vi "Helper - Find All Substring Locations.vi"(10 "search string":string, 11 "input string":string) -> (3 "Locations":i32[](array[numeric]))   [LabVIEW 2011]
doc: "Finds ALL instances of the search string in the input string and outputs the locations in an array."
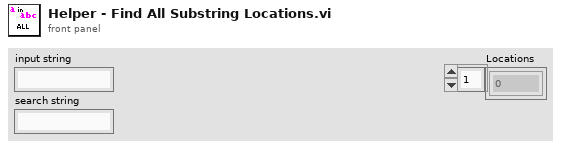
[diagram p1: front panel]
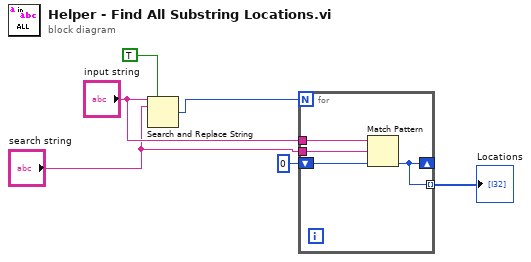
[diagram p0: block diagram]
diagram:
  n1 = Search and Replace String(replace all?=TRUE ("replace all? (F)"), input string="input string", search string="search string") -> (number of replacements=w6:i32)  [unwired: 5 in, 3 out]
  n2 = for {
    N: w6 -> [_]
    tunnel: "search string" -> [w9]
    tunnel: "input string" -> [w10]
    shift-right: [w7] -> _
    shift-left: 0 ("offset past match") -> [w8]
    tunnel: [w7] -> w2 mode=indexing
    n3 = Match Pattern(string=w10, regular expression=w9, offset (0)=w8) -> (offset past match=w7:i32)  [unwired: 3 out]
  }
  "Locations" <- w2
